vi "Filtra_Tag_prioridades_server.vi"(11 "padrao_TAGS_prioridade_client":T1) -> (3 "TAGs prioridade":string[](array[string]))   [LabVIEW 2019]
uses:
  padrao_TAGS_prioridades_client.ctl
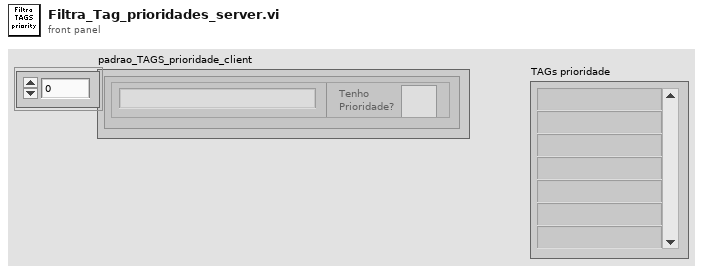
[diagram p1: front panel]
types:
  T1 = typedef "padrao_TAGS_prioridades_client.ctl" = cluster{"TAG":string, "Tenho\nPrioridade?":bool}[]
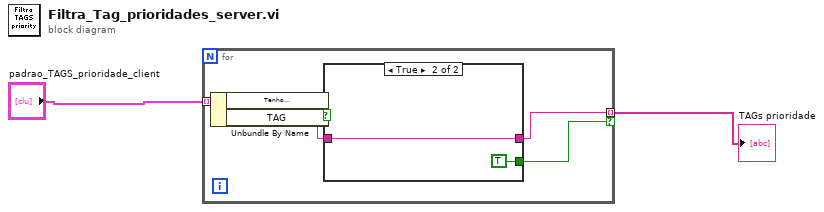
[diagram p0: block diagram]
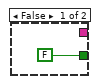
[diagram p2: hidden frame]
diagram:
  n1 = for {
    tunnel: "padrao_TAGS_prioridade_client" -> [w6] mode=indexing
    tunnel: [w5] -> w1 mode=indexing if=w4
    n2 = Unbundle By Name(w6) -> ("Tenho\nPrioridade?"=w7:bool, "TAG"=w3:string)
    n3 = case shown="True" w7 {
      tunnel: w3 -> [_ w10]
      tunnel: [_ w10] -> w5
      tunnel: [FALSE TRUE] -> w4
      frame False {
      }
      frame True {
      }
    }
  }
  "TAGs prioridade" <- w1
